vi "Joystickfunctionfull L (SubVI).vi"   [LabVIEW 2012]
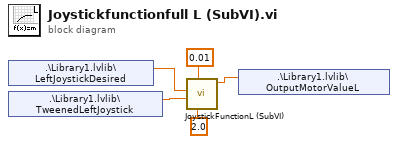
[diagram p0: block diagram]
diagram:
  n1 = shared-variable ".\\Library1.lvlib\\LeftJoystickDesired"() -> (w4:dbl)  [unwired: 1 in, 1 out]
  n2 = shared-variable ".\\Library1.lvlib\\TweenedLeftJoystick"() -> (w5:dbl)  [unwired: 1 in, 1 out]
  n3 = call "JoystickFunctionL (SubVI).vi"("TimeToReachSpeed"=2.0 ("y"), "DeltaT"=0.01 ("y"), "TweenedSpeed"=w5, "DesiredSpeed"=w4) -> ("OutputMotorValueL"=w3:dbl)  [unwired: 7 in]
  n4 = shared-variable ".\\Library1.lvlib\\OutputMotorValueL"(w3) -> ()  [unwired: 1 in, 1 out]
